vi "GetXmlString.vi"(8 "error in":errorcluster caption="错误输入（无错误）", 11 "PanelRootNode 输入":refnum<class "PanelRootNode.lvclass"> caption="DNL_LabVIEW Object in") -> (0 "error out":errorcluster caption="错误输出", 2 "XML":string, 3 "PanelRootNode 输出":refnum<class "PanelRootNode.lvclass"> caption="DNL_LabVIEW Object out")   [LabVIEW 2016, in "PanelRootNode.lvclass"]
uses:
  PanelRootNode.lvclass
  <vilib>/xml/Close Reference(Node).vi
  <resource>/objmgr/DOMUserDefRef.rc
  <vilib>/xml/NI_XML.lvlib
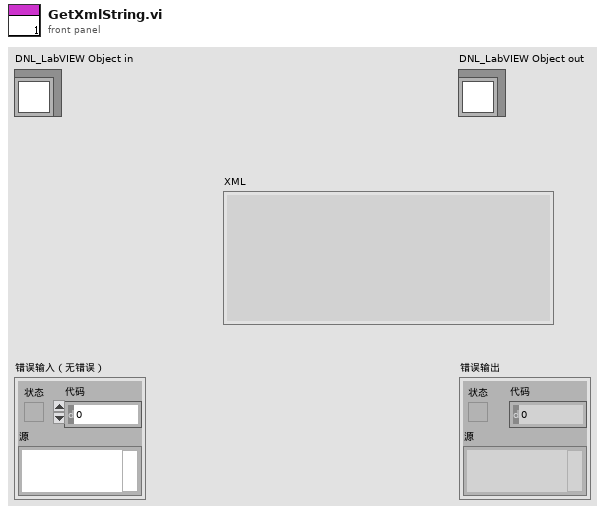
[diagram p1: front panel]
types:
  T1 = cluster{"DOM Ref":refnum<k20>, "Element Ref":refnum<k20>}
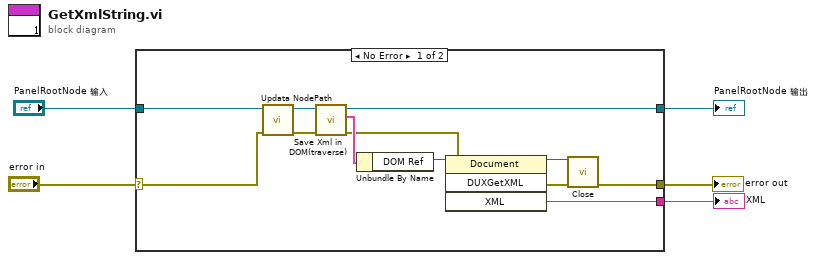
[diagram p0: block diagram]
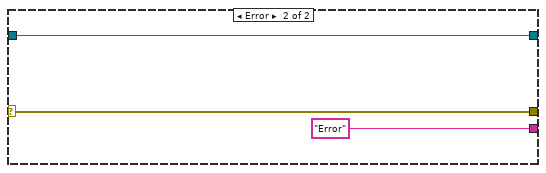
[diagram p2: hidden frame]
diagram:
  n1 = case shown="No Error" "error in" {
    selector: "error in" -> [w8 w20]
    tunnel: [w7 w20] -> w4
    tunnel: [w14 w19] -> w2
    tunnel: "PanelRootNode 输入" -> [w15 w19]
    tunnel: [w6 "Error" ("XML")] -> w1
    frame No Error {
      n2 = call-dynamic "Updata NodePath.vi"("error in"=w8, "PanelLinkNode 输入"=w15) -> ("error out"=w17:errorcluster, "PanelLinkNode 输出"=w16:refnum<class "PanelRootNode.lvclass">)  [unwired: 8 in]
      n3 = call "Save Xml in DOM(traverse).vi"("error in"=w17, "PanelRootNode.lvclass"=w16) -> ("error out"=w10:errorcluster, "Data out"=w13:T1, "PanelRootNode out"=w14:refnum<class "PanelRootNode.lvclass">)  [unwired: 7 in]
      n4 = Unbundle By Name(w13) -> ("DOM Ref"=w12:refnum<k20>)
      n5 = invoke class="Document" method="DUXGetXML"(reference=w12, error in=w10) -> (reference out=w11:refnum<k20>, error out=w9:errorcluster, "XML"=w6:string)  [unwired: 2 in, 1 out]
      n6 = call-poly <vilib>:"Close.vi"("error in (no error)"=w9, "node"=w11) -> ("error out"=w7:errorcluster)  [unwired: 7 in]
    }
    frame Error {
    }
  }
  "error out" <- w4
  "PanelRootNode 输出" <- w2
  "XML" <- w1
